vi "Read Instrument Handle.vi"(8 "error in (no error)":errorcluster, 11 "IVI_DMM in":refnum<class "IVI_DMM.lvclass">) -> (0 "error out":errorcluster, 2 "Instrument Handle":refnum<k15>, 3 "IVI_DMM out":refnum<class "IVI_DMM.lvclass">)   [LabVIEW 2016, in "IVI_DMM.lvlib" / "IVI_DMM.lvclass"]
doc: "Read instrument handle."
uses:
  IVI_DMM.lvclass
  IVI_DMM.lvclass/IVI_DMM.ctl
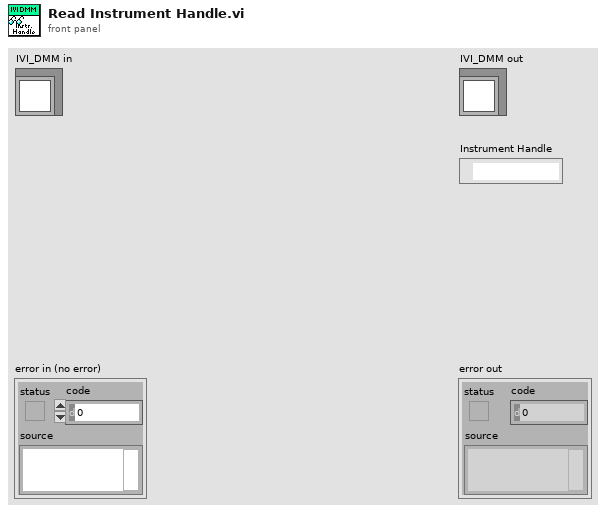
[diagram p1: front panel]
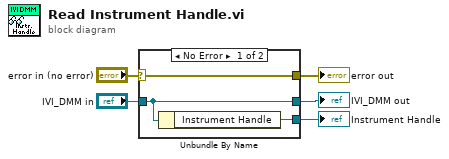
[diagram p0: block diagram]
diagram:
  n1 = case shown="No Error" "error in (no error)" {
    selector: "error in (no error)" -> [w8 w9]
    tunnel: [w8 w9] -> w4
    tunnel: [w7 w10] -> w2
    tunnel: "IVI_DMM in" -> [w7 w10]
    tunnel: [w6 _] -> w1
    frame No Error {
      n2 = Unbundle By Name(w7) -> ("Instrument Handle"=w6:refnum<k15>)
    }
    frame Error {
    }
  }
  "error out" <- w4
  "IVI_DMM out" <- w2
  "Instrument Handle" <- w1
